vi "Global 3.vi"() -> ()   [LabVIEW 2013]
panel:
  out "Virus C":dbl(slide) scale=0.0..80.0
  out "Virus B":dbl(slide) scale=0.0..80.0
  out "Virus A":dbl(slide) scale=0.0..80.0
  out "Water":dbl(slide) scale=0.0..50.0
  out "Classifier material":dbl(slide) scale=0.0..25.0
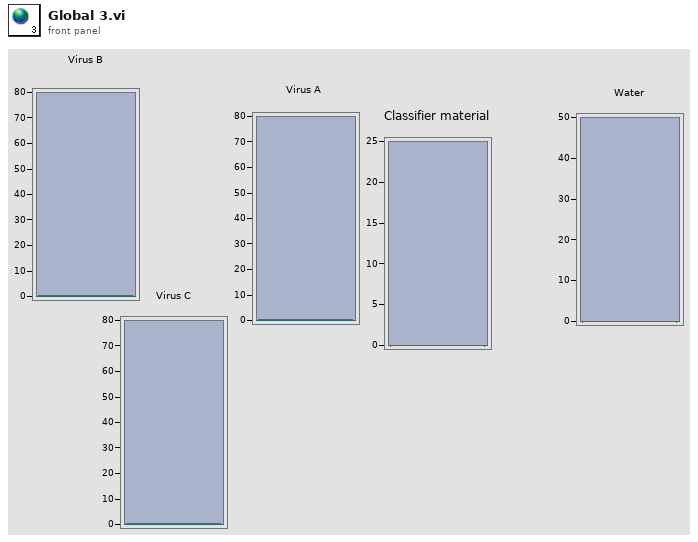
[diagram p1: front panel]
diagram:
